vi "Write Port.vi"(8 "error in":errorcluster, 10 "port":u16, 11 "TCP slave in":refnum<class "TCP Slave.lvclass">) -> (0 "error out":errorcluster, 3 "TCP slave out":refnum<class "TCP Slave.lvclass">)   [LabVIEW 2021, in "TCP Slave.lvclass"]
doc: "Property accessor for the TCP port."
uses:
  TCP Slave.lvclass
  TCP Slave.lvclass/TCP Slave.ctl
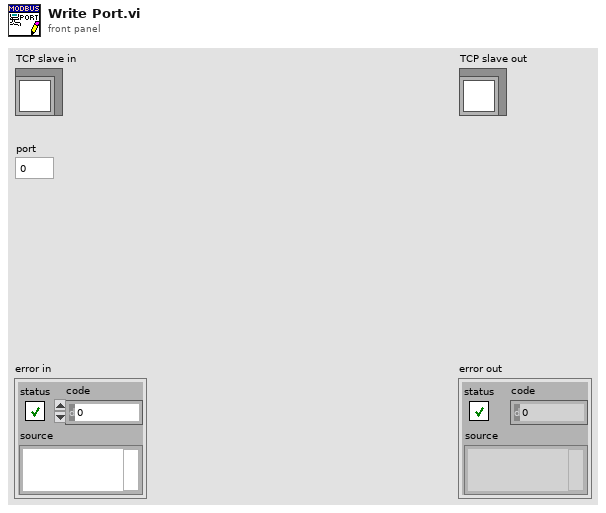
[diagram p1: front panel]
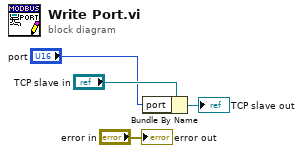
[diagram p0: block diagram]
diagram:
  n1 = Bundle By Name(cluster="TCP slave in", "port"="port") -> (→"TCP slave out":refnum<class "TCP Slave.lvclass">)
  "error out" <- "error in"
